vi "sv_UFF58 Read Channel Data.vi"(0 "function refnum":refnum<k20>, 5 "channel to read":enum16{"X", "Y Real", "Y Imaginary"}(ring), 11 "error in (no error)":errorcluster) -> (4 "dup function refnum":refnum<k20>, 6 "data":dbl[](array[numeric]), 15 "error out":errorcluster)   [LabVIEW 2017, in "SoundVib_UFF58.lvlib"]
doc: "This VI reads the <B>data</B> contained in the given <B>channel to read</B> for the input <B>function refnum</B>."
uses:
  <vilib>/addons/Sound and Vibration/svt_UFF58/SoundVib_UFF58.lvlib
  <vilib>/Platform/storage/Storage.llb/Get Property (Storage Refnums).vi
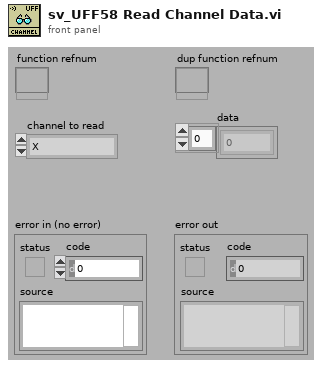
[diagram p1: front panel]
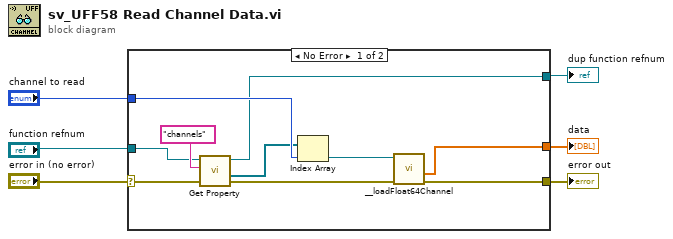
[diagram p0: block diagram]
diagram:
  n1 = case shown="No Error" "error in (no error)" {
    selector: "error in (no error)" -> [w9 w18]
    tunnel: [w16 w18] -> w6
    tunnel: [w15 _] -> w5
    tunnel: "channel to read" -> [w14 _]
    tunnel: [w11 w17] -> w1
    tunnel: "function refnum" -> [w10 w17]
    frame No Error {
      n2 = call-poly <vilib>:"Get Property.vi"("error in (no error)"=w9, "Property name"="channels", "storage refnum"=w10) -> ("error out"=w8:errorcluster, "Value"=w12:refnum<k20>[], "storage refnum out"=w11:refnum<k20>)  [unwired: 6 in]
      n3 = Index Array(array=w12, index=w14) -> (element=w7:refnum<k20>)
      n4 = call <vilib>:"__loadFloat64Channel.vi"("error in (no error)"=w8, "Data object in"=w7) -> ("error out"=w16:errorcluster, "Values"=w15:dbl[])  [unwired: 2 in, 2 out]
    }
    frame Error {
    }
  }
  "error out" <- w6
  "data" <- w5
  "dup function refnum" <- w1
